vi "Merge_Status_Clusters.vi"(1 "Status Cluster 2":T1, 2 "Status Cluster 1":T1) -> (0 "Status Cluster Out":T1)   [LabVIEW 2010]
uses:
  Status_Cluster.ctl
  Multi_Run_Status.ctl
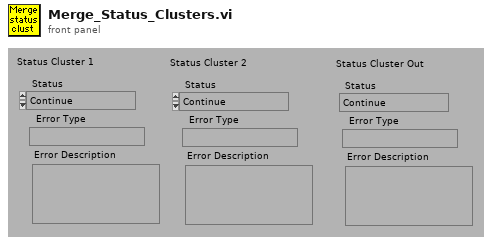
[diagram p1: front panel]
types:
  T1 = typedef "Status_Cluster.ctl" = cluster{"Status":T2, "Error Type":string, "Error Description":string}
  T2 = typedef "Multi_Run_Status.ctl" = enum16{"Continue", "Jump to Next Point", "Jump to Next Row", "Jump To Fall Back", "Terminate Run"}
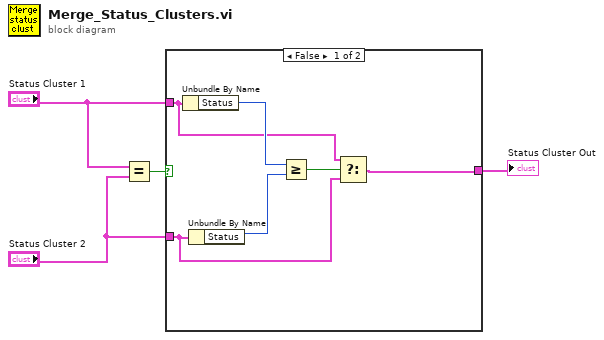
[diagram p0: block diagram]
diagram:
  n1 = Equal?(x="Status Cluster 1", y="Status Cluster 2") -> (x = y?=w4:bool)
  n2 = case shown="False" w4 {
    tunnel: [w5 w11] -> w3
    tunnel: "Status Cluster 1" -> [w7 w11]
    tunnel: "Status Cluster 2" -> [w6 _]
    frame False {
      n3 = Unbundle By Name(w7) -> ("Status"=w10:T2)
      n4 = Unbundle By Name(w6) -> ("Status"=w9:T2)
      n5 = Greater Or Equal?(x=w10, y=w9) -> (x >= y?=w8:bool)
      n6 = Select(t=w7, s=w8, f=w6) -> (s? t:f=w5:T1)
    }
    frame True {
    }
  }
  "Status Cluster Out" <- w3
